vi "get Decon Mat Size LV.vi"(6 "iRF_array":dbl[](array[numeric]), 8 "error in (no error)":errorcluster, 9 "alpha":dbl, 10 "dataLength":u64, 11 "laguerreOrder":u64) -> (0 "error out":errorcluster, 3 "daat Matrix Szie":T1)   [LabVIEW 2024, in "LaguerreDeconLib.lvlib"]
doc: "extern \"C\" DECONLIBRARY_API void getDeconMatSizeLV(const unsigned long long laguerreOrder, const unsigned long long dataLength, const double alpha, const double* iRF_array, const unsigned long long iRF_length,\n unsigned long long* rows1, unsigned long long* cols1,\n unsigned long long* rows2, unsigned long long* cols2,\n unsigned long long* rows3, unsigned long long* cols3,\n unsigned long long* rows4, unsigned long long* cols4,\n unsigned long long* rows5, unsigned long long* cols5);"
uses:
  LaguerreDeconLib.lvlib
  LaguerreDeconDLL.dll
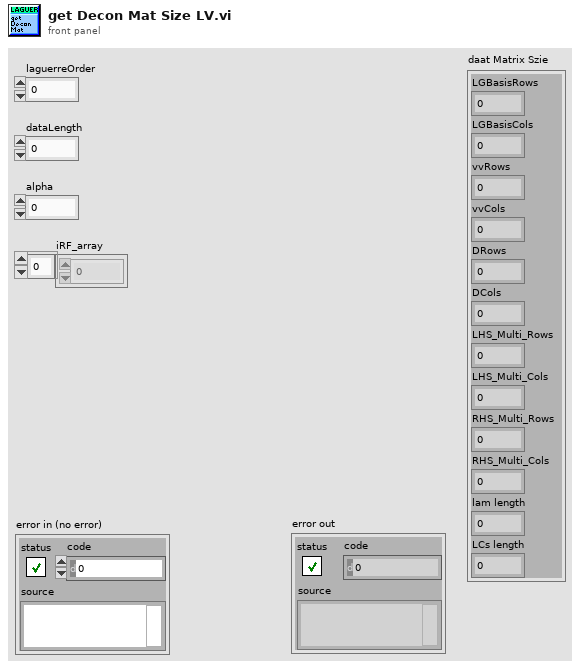
[diagram p1: front panel]
types:
  T1 = cluster{"LGBasisRows":u32, "LGBasisCols":u32, "vvRows":u32, "vvCols":u32, "DRows":u32, "DCols":u32, "LHS_Multi_Rows":u32, "LHS_Multi_Cols":u32, "RHS_Multi_Rows":u32, "RHS_Multi_Cols":u32, "lam length":u32, "LCs length":u32}
  T2 = cluster{"LGBasisRows":u64, "LGBasisCols":u64, "vvRows":u64, "vvCols":u64, "DRows":u64, "DCols":u64, "LHS_Multi_Rows":u64, "LHS_Multi_Cols":u64, "RHS_Multi_Rows":u64, "RHS_Multi_Cols":u64, "lam length":u64, "LCs length":u64}
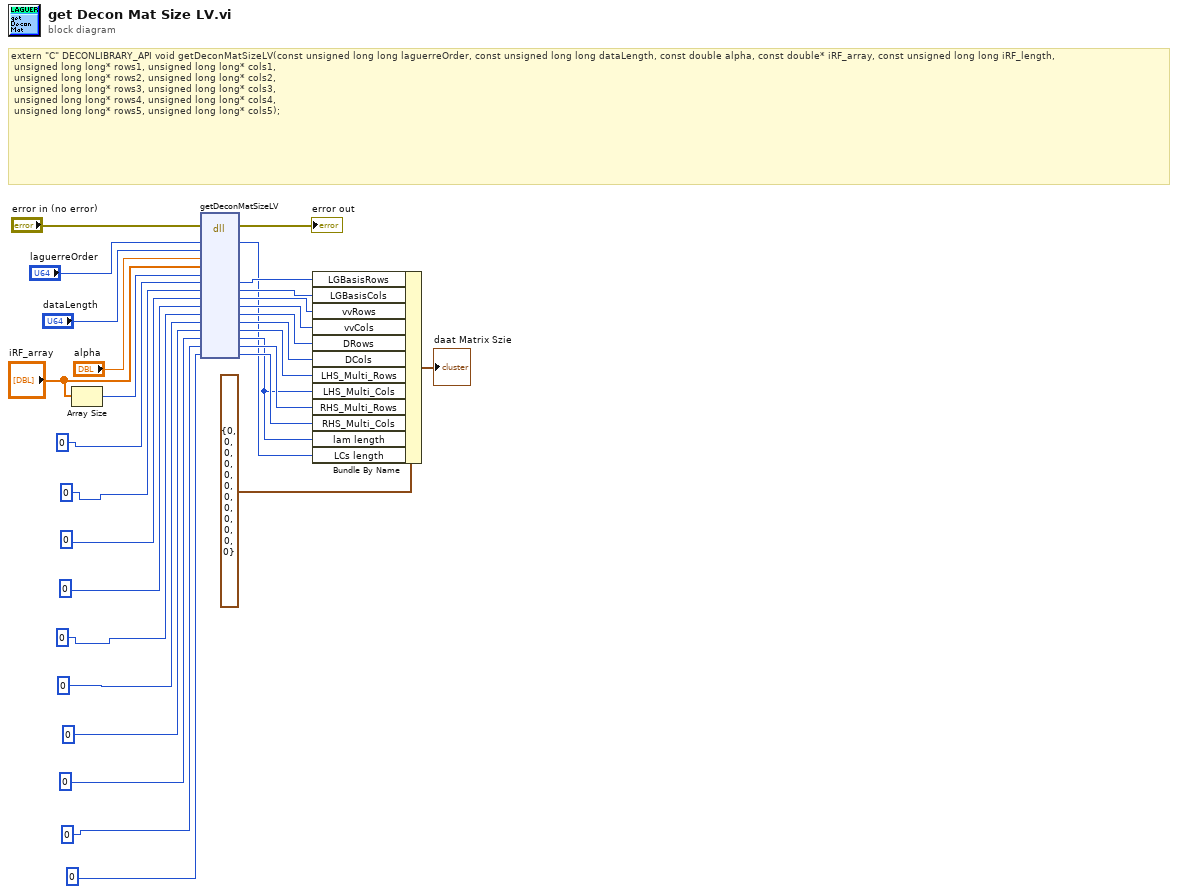
[diagram p0: block diagram]
diagram:
  # "extern \"C\" DECONLIBRARY_API void getDeconMatSizeLV(const unsigned long long laguerreOrder, const unsigned long long dataLength, const double alpha, const double* iRF_array, const unsigned long long iRF_length,\n\tunsigned long long* rows1, unsigned long long* cols1,\n\tunsigned long long* rows2, unsigned long long* cols2,\n\tunsigned long long* rows3, unsigned long long* cols3,\n\tunsigned long long* rows4, unsigned long long* cols4,\n\tunsigned long long* rows5, unsigned long long* cols5);"
  n1 = Array Size(array="iRF_array") -> (size(s)=w15:i32)
  n2 = dll-call lib="C:/Users/MarcuLab/Desktop/V6 APD LV/V6 APD LV/LaguerreDeconLib/LaguerreDeconDLL.dll" fn="getDeconMatSizeLV"(error in="error in (no error)", "laguerreOrder"="laguerreOrder", "dataLength"="dataLength", "alpha"="alpha", "iRF_array"="iRF_array", "iRF_length"=w15, "LGBasisRows"=u64 0, "LGBasisCols"=u64 0, "vvRows"=u64 0, "vvCols"=u64 0, "DRows"=u64 0, "DCols"=u64 0, "LHS_Multi_Rows"=u64 0, "LHS_Multi_Cols"=u64 0, "RHS_Multi_Rows"=u64 0, "RHS_Multi_Cols"=u64 0) -> (error out=→"error out":errorcluster, "laguerreOrder"=w11:u64, "LGBasisRows"=w25:u64, "LGBasisCols"=w24:u64, "vvRows"=w23:u64, "vvCols"=w22:u64, "DRows"=w21:u64, "DCols"=w20:u64, "LHS_Multi_Rows"=w19:u64, "LHS_Multi_Cols"=w12:u64, "RHS_Multi_Rows"=w18:u64, "RHS_Multi_Cols"=w17:u64)  [unwired: 7 in, 1 out]
  n3 = Bundle By Name(cluster=T2 {"LGBasisRows"=0, "LGBasisCols"=0, "vvRows"=0, "vvCols"=0, "DRows"=0, "DCols"=0, "LHS_Multi_Rows"=0, "LHS_Multi_Cols"=0, "RHS_Multi_Rows"=0, "RHS_Multi_Cols"=0, "lam length"=0, "LCs length"=0} ("daat Matrix Szie"), "LGBasisRows"=w25, "LGBasisCols"=w24, "vvRows"=w23, "vvCols"=w22, "DRows"=w21, "DCols"=w20, "LHS_Multi_Rows"=w19, "LHS_Multi_Cols"=w12, "RHS_Multi_Rows"=w18, "RHS_Multi_Cols"=w17, "lam length"=w12, "LCs length"=w11) -> (→"daat Matrix Szie":T2)
